vi "Load from Include File.vi"(8 "error in (no error)":errorcluster, 11 "Coverage Report in":refnum<class "Coverage Report.lvclass">) -> (0 "error out":errorcluster, 3 "Coverage Report out":refnum<class "Coverage Report.lvclass">)   [LabVIEW 2020, in "Coverage Report.lvclass"]
uses:
  Coverage Report.lvclass
  Coverage Report.lvclass/Coverage Report.ctl
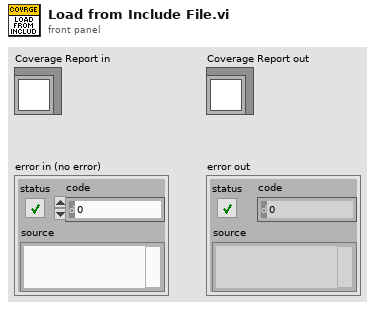
[diagram p1: front panel]
types:
  T1 = enum16{"open", "replace", "create", "open or create", "replace or create", "replace or create with confirmation"}
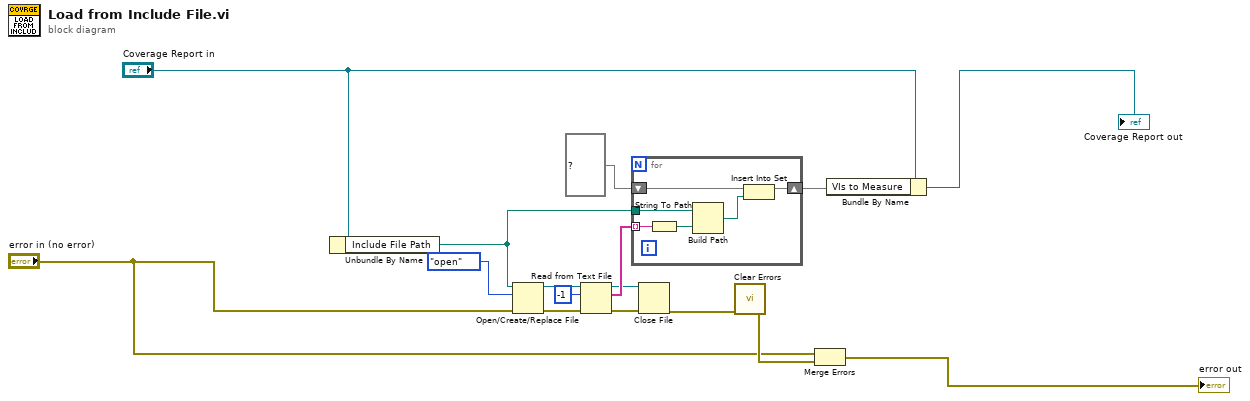
[diagram p0: block diagram]
diagram:
  n1 = Unbundle By Name("Coverage Report in") -> ("Include File Path"=w16:path)
  n2 = Open/Create/Replace File(file path (use dialog)=w16, error in="error in (no error)", operation (0:open)=T1."open") -> (refnum out=w5:refnum<file>, error out=w2:errorcluster)  [unwired: 3 in, 1 out]
  n3 = Read from Text File(file (use dialog)=w5, count=-1, error in=w2) -> (refnum out=w6:refnum<file>, text=w10:string[], error out=w4:errorcluster)  [unwired: 1 in, 1 out]
  n4 = for {
    shift-right: [w21] -> w11
    shift-left: set{path} {} ("VIs to Measure") -> [w22]
    tunnel: w10 -> [w20] mode=indexing
    tunnel: w16 -> [w17]
    n5 = String To Path(string=w20) -> (path=w18:path)
    n6 = Build Path(base path=w17, name or relative path=w18) -> (appended path=w19:path)
    n7 = Insert Into Set(10:w19, 11:w22) -> (3:w21:set{path})  [unwired: 1 out]
  }
  n8 = Close File(refnum=w6, error in=w4) -> (error out=w7:errorcluster)  [unwired: 1 out]
  n9 = call <vilib>:"Clear Errors.vi"("error in (no error)"=w7) -> ("error out"=w15:errorcluster)  [unwired: 5 in, 1 out]
  n10 = Merge Errors("error in (no error)", w15) -> (→"error out":errorcluster)
  n11 = Bundle By Name(cluster="Coverage Report in", "VIs to Measure"=w11) -> (→"Coverage Report out":refnum<class "Coverage Report.lvclass">)
